vi "maxVelToBreak.vi"(0 "Game in":refnum<class "Game.lvclass">, 1 "desired_vel":dbl, 2 "delta":dbl, 3 "est_vel":dbl, 5 "error in (no error)":errorcluster, 6 "array":dbl[][](array[numeric]), 7 "dist":dbl, 9 "v_max":dbl) -> (14 "Game out":refnum<class "Game.lvclass">, 16 "vel":dbl, 19 "error out":errorcluster)   [LabVIEW 2023, in "Game.lvclass"]
uses:
  Game.lvclass
  <vilib>/Analysis/1siggen.llb/Ramp Pattern by Delta.vi
  <vilib>/Analysis/NI_AALBase.lvlib
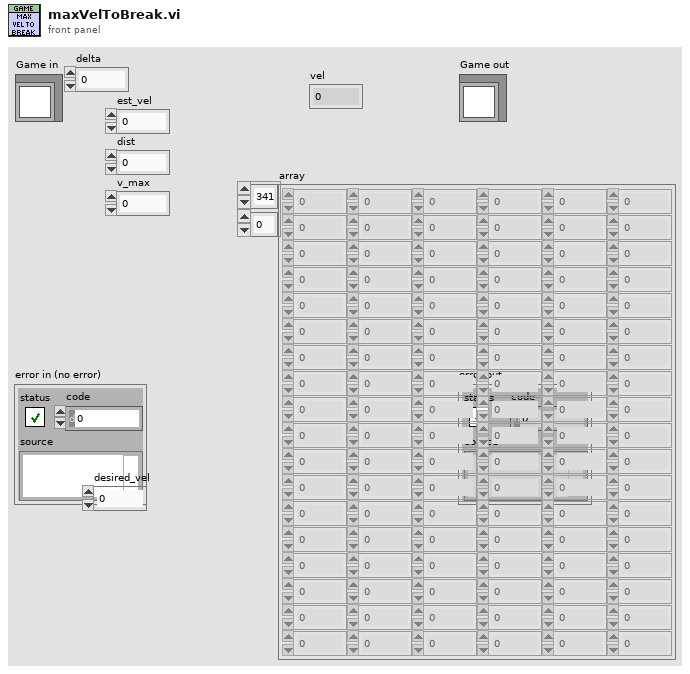
[diagram p1: front panel]
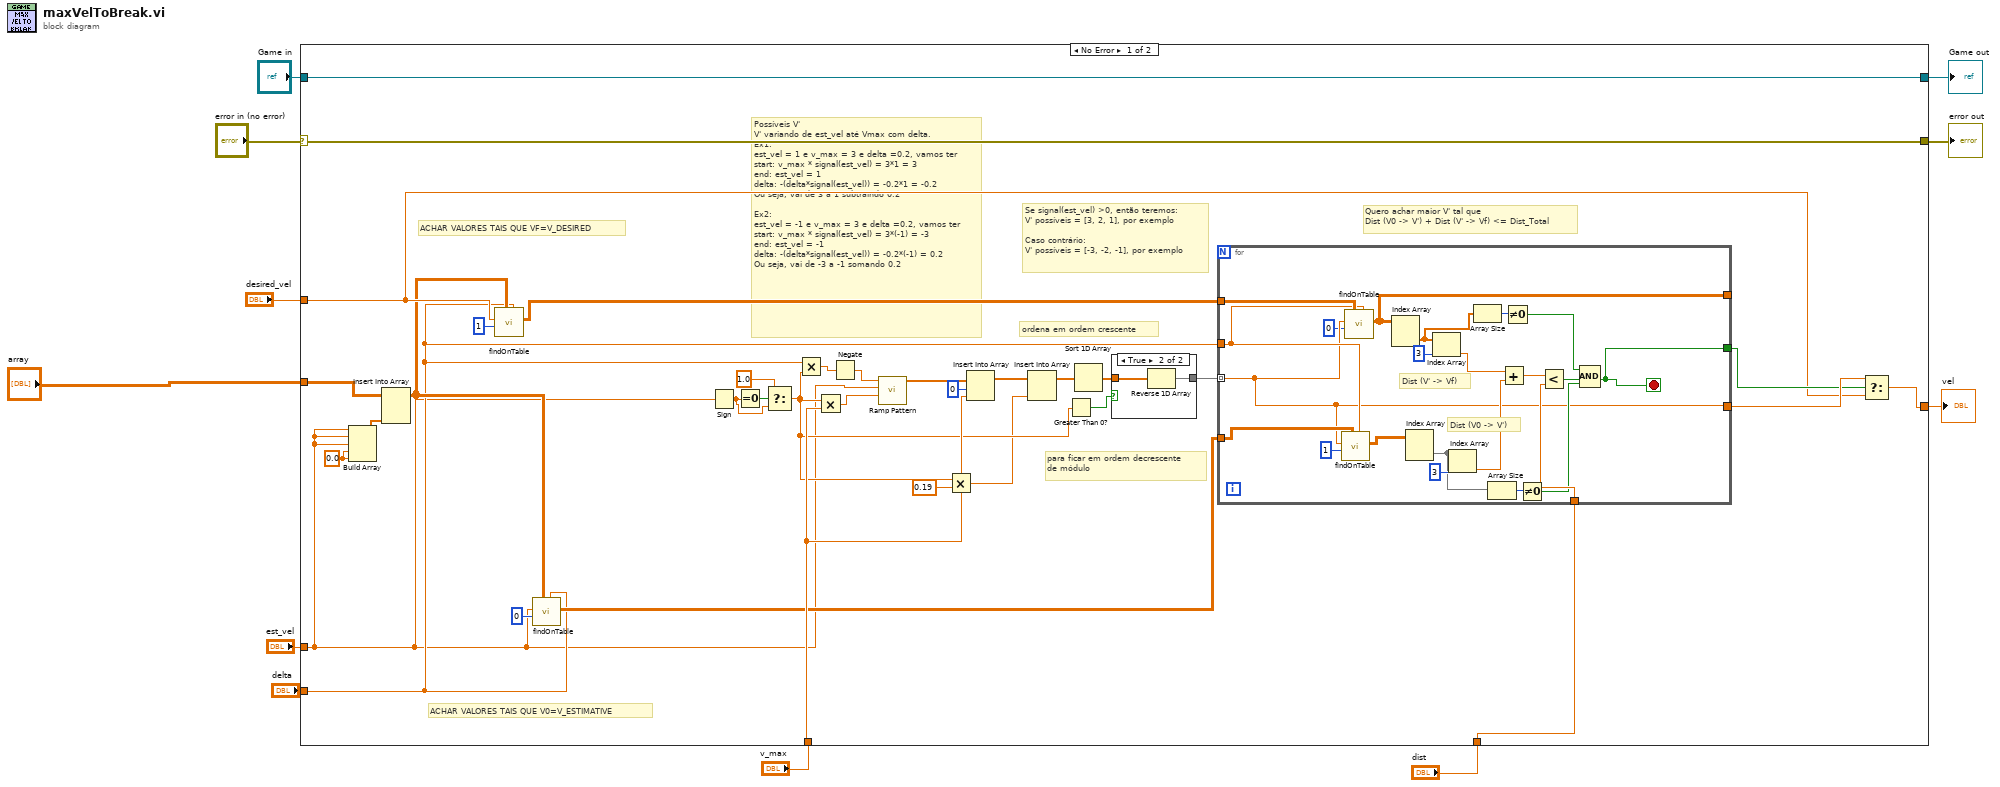
[diagram p0: block diagram]
diagram:
  n1 = case shown="No Error" "error in (no error)" {
    selector: "error in (no error)" -> [w44 w72]
    tunnel: [w44 w72] -> w10
    tunnel: [w45 w71] -> w8
    tunnel: "Game in" -> [w45 w71]
    tunnel: "array" -> [w33 _]
    tunnel: "desired_vel" -> [w28 _]
    tunnel: "delta" -> [w24 _]
    tunnel: "est_vel" -> [w13 _]
    tunnel: "dist" -> [w37 _]
    tunnel: "v_max" -> [w34 _]
    tunnel: [w39 _] -> w2
    frame No Error {
      w30 = 0.0 ("element")
      # "Se signal(est_vel) >0, então teremos:\nV' possíveis = [3, 2, 1], por exemplo\n\nCaso contrário:\nV' possíveis = [-3, -2, -1], por exemplo"
      # "para ficar em ordem decrescente\nde módulo"
      # "ordena em ordem crescente"
      # "Possíveis V'\nV' variando de est_vel até Vmax com delta.\nEx1:\nest_vel = 1 e v_max = 3 e delta =0.2, vamos ter\nstart: v_max * signal(est_vel) = 3*1 = 3\nend: est_vel = 1\ndelta: -(delta*signal(est_vel)) = -0.2*1 = -0.2\nOu seja, vai de 3 a 1 subtraindo 0.2\n\nEx2:\nest_vel = -1 e v_max = 3 e delta =0.2, vamos ter\nstart: v_max * signal(est_vel) = 3*(-1) = -3\nend: est_vel = -1\ndelta: -(delta*signal(est_vel)) = -0.2*(-1) = 0.2\nOu seja, vai de -3 a -1 somando 0.2"
      # "Quero achar maior V' tal que\nDist (V0 -> V') + Dist (V' -> Vf) <= Dist_Total"
      # "ACHAR VALORES TAIS QUE V0=V_ESTIMATIVE"
      # "ACHAR VALORES TAIS QUE VF=V_DESIRED"
      n2 = Build Array(w13, w13, w13, w30, w30) -> (w32:dbl[])
      n3 = Insert Into Array(array=w33, new element=w32) -> (w25:dbl[][])  [unwired: 2 in]
      n4 = call "findOnTable.vi"("delta"=w24, "table"=w25, "column"=1, "key"=w28) -> ("search_results"=w29:dbl[][])  [unwired: 5 in, 2 out]
      n5 = call "findOnTable.vi"("delta"=w24, "table"=w25, "column"=0, "key"=w13) -> ("search_results"=w26:dbl[][])  [unwired: 5 in, 2 out]
      n6 = Sign(1:w13) -> (0:w21:dbl)
      n7 = Equal To 0?(x=w21) -> (x = 0?=w22:bool)
      n8 = Select(t=1.0, s=w22, f=w21) -> (s? t:f=w15:dbl)
      n9 = Multiply(x=w24, y=w15) -> (x*y=w41:dbl)
      n10 = Multiply(x=w15, y=w34) -> (x*y=w42:dbl)
      n11 = Negate(x=w41) -> (-x=w43:dbl)
      n12 = call-poly <vilib>:"Ramp Pattern.vi"("start"=w42, "end"=w13, "delta"=w43) -> ("Ramp Pattern"=w36:dbl[])  [unwired: 6 in, 2 out]
      n13 = Multiply(x=w15, y=0.19) -> (x*y=w14:dbl)
      n14 = Insert Into Array(array=w36, index=0, new element=w34) -> (w31:dbl[])
      n15 = Insert Into Array(array=w31, new element=w14) -> (w18:dbl[])  [unwired: 1 in]
      n16 = Greater Than 0?(x=w15) -> (x > 0?=w16:bool)
      n17 = Sort 1D Array(array=w18) -> (sorted array=w19:dbl[])
      n18 = case shown="True" w16 {
        tunnel: w19 -> [w46 w48]
        tunnel: [w46 w47] -> w17
        frame False {
        }
        frame True {
          n19 = Reverse 1D Array(array=w48) -> (reversed array=w47:dbl[])
        }
      }
      n20 = for {
        tunnel: w17 -> [w50] mode=indexing
        tunnel: w29 -> [w52]
        tunnel: w26 -> [w55]
        tunnel: w24 -> [w51]
        tunnel: w37 -> [w70]
        tunnel: [w50] -> w40
        tunnel: [w59] -> w38
        tunnel: [w53] -> _
        stop <- w59 stop-if-true
        # "Dist (V' -> Vf)"
        # "Dist (V0 -> V')"
        n21 = call "findOnTable.vi"("delta"=w51, "table"=w55, "column"=1, "key"=w50) -> ("search_results"=w56:dbl[][])  [unwired: 5 in, 2 out]
        n22 = call "findOnTable.vi"("delta"=w51, "table"=w52, "column"=0, "key"=w50) -> ("search_results"=w53:dbl[][])  [unwired: 5 in, 2 out]
        n23 = Index Array(array=w53) -> (element=w64:dbl[])  [unwired: 2 in]
        n24 = Index Array(array=w56) -> (element=w58:dbl[])  [unwired: 2 in]
        n25 = Index Array(array=w64, index=3) -> (element=w66:dbl)
        n26 = Index Array(array=w58, index=3) -> (element=w68:dbl)
        n27 = Array Size(array=w64) -> (size(s)=w63:i32)
        n28 = Array Size(array=w58) -> (size(s)=w62:i32)
        n29 = Add(x=w66, y=w68) -> (x+y=w65:dbl)
        n30 = Not Equal To 0?(x=w63) -> (x != 0?=w57:bool)
        n31 = Not Equal To 0?(x=w62) -> (x != 0?=w60:bool)
        n32 = Less?(x=w65, y=w70) -> (x < y?=w61:bool)
        n33 = Compound Arithmetic op=AND(w57, w61, w60) -> (w59:bool)
      }
      n34 = Select(t=w40, s=w38, f=w28) -> (s? t:f=w39:dbl)
    }
    frame Error {
    }
  }
  "error out" <- w10
  "Game out" <- w8
  "vel" <- w2
